vi "Close Supply.vi"(0 "Supply Line Handle in":refnum<k15>, 11 "error in (no error)":errorcluster) -> (15 "error out":errorcluster)   [LabVIEW 2016, in "Supply.lvlib"]
uses:
  Supply.lvlib
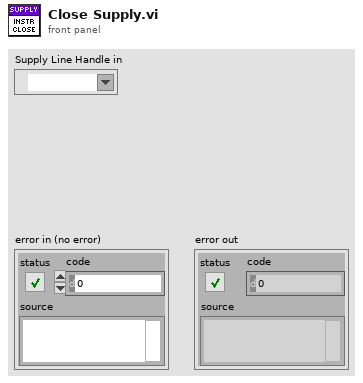
[diagram p1: front panel]
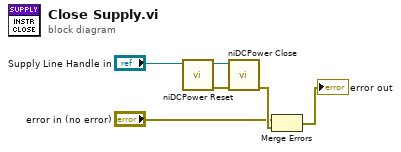
[diagram p0: block diagram]
diagram:
  n1 = call <instrlib>:"niDCPower Reset.vi"("instrument handle"="Supply Line Handle in") -> ("error out"=w4:errorcluster, "instrument handle out"=w6:refnum<k15>)  [unwired: 9 in]
  n2 = call <instrlib>:"niDCPower Close.vi"("error in (no error)"=w4, "instrument handle"=w6) -> ("error out"=w3:errorcluster)  [unwired: 9 in]
  n3 = Merge Errors("error in (no error)", w3) -> (→"error out":errorcluster)
